vi "03_dosing.vi"() -> ()   [LabVIEW 2024]
uses:
  <vilib>/Utility/error.llb/DialogType.ctl
  <vilib>/Waveform/WDTOps.llb/WDT Waveform to XY Pairs DBL.vi
  <instrlib>/Tektronix DMM40x0 Series/Tektronix DMM40x0 Series.lvlib
panel:
  out "error out":errorcluster
  out "error out 2":errorcluster caption="error out"
  out "STABLE":bool
  in  "Serial Communication":T1={"Baud Rate"=9600, "Parity"=0, "Data Bits"=8, "Stop Bits"=10, "Flow Control"=0} {"Flow Control" items=["None", "XON/XOFF", "RTS/CTS", "XON/XOFF & RTS/CTS", "DTR/DSR", "XON/XOFF & DTR/DSR"]; "Stop Bits" items=["1.0"=10, "1.5"=15, "2.0"=20]; "Data Bits" items=["7"=7, "8"=8]; "Parity" items=["None", "Odd", "Even", "Mark", "Space"]; "Baud Rate" items=["300"=300, "600"=600, "1200"=1200, "2400"=2400, "4800"=4800, "9600"=9600, "19200"=19200]}
  in  "COM PORT (COM2)":refnum<visa-resource-name>
  out "Stability threshold":dbl format="%#_13g"
  out "Waveform Graph":dbl[](graph)
  out "XY pairs":cluster{"x":timestamp, "y":dbl}[](array[cluster]) {"y" format="%0.2f"}
  # "Voltmeter Serial Configuration"
  # "DEFAULT SETTINGS:\n\nTimeout (10000 ms)\nTrigger Count (5000)\nSample Count (1)\n\n****DC VOLTAGE***"
  # "Voltmeter Stability"
  # "0 - Stability threshold not met\n1 - Stability threshold met\n\n\n\n*stability (+/-0.05 mV) of last 15 pts"
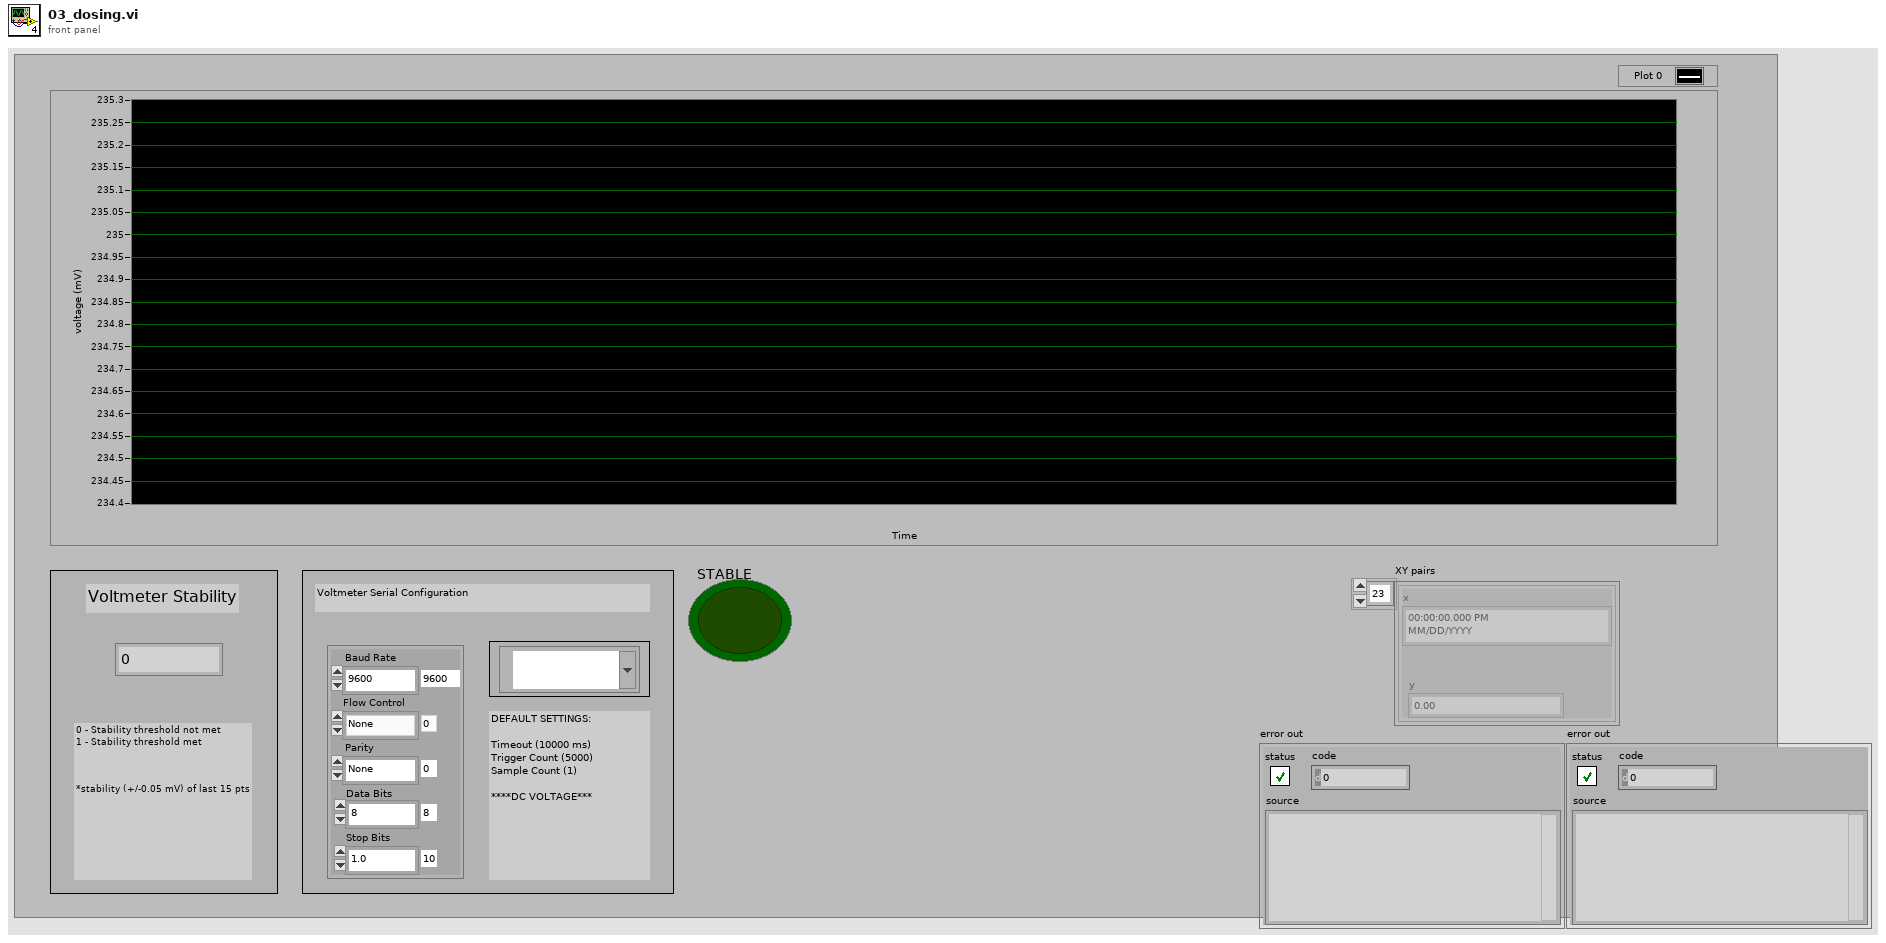
[diagram p1: front panel]
types:
  T1 = cluster{"Baud Rate":u32, "Parity":u16, "Data Bits":u16, "Stop Bits":u16, "Flow Control":u16}
  T2 = typedef "DialogType.ctl" = u16
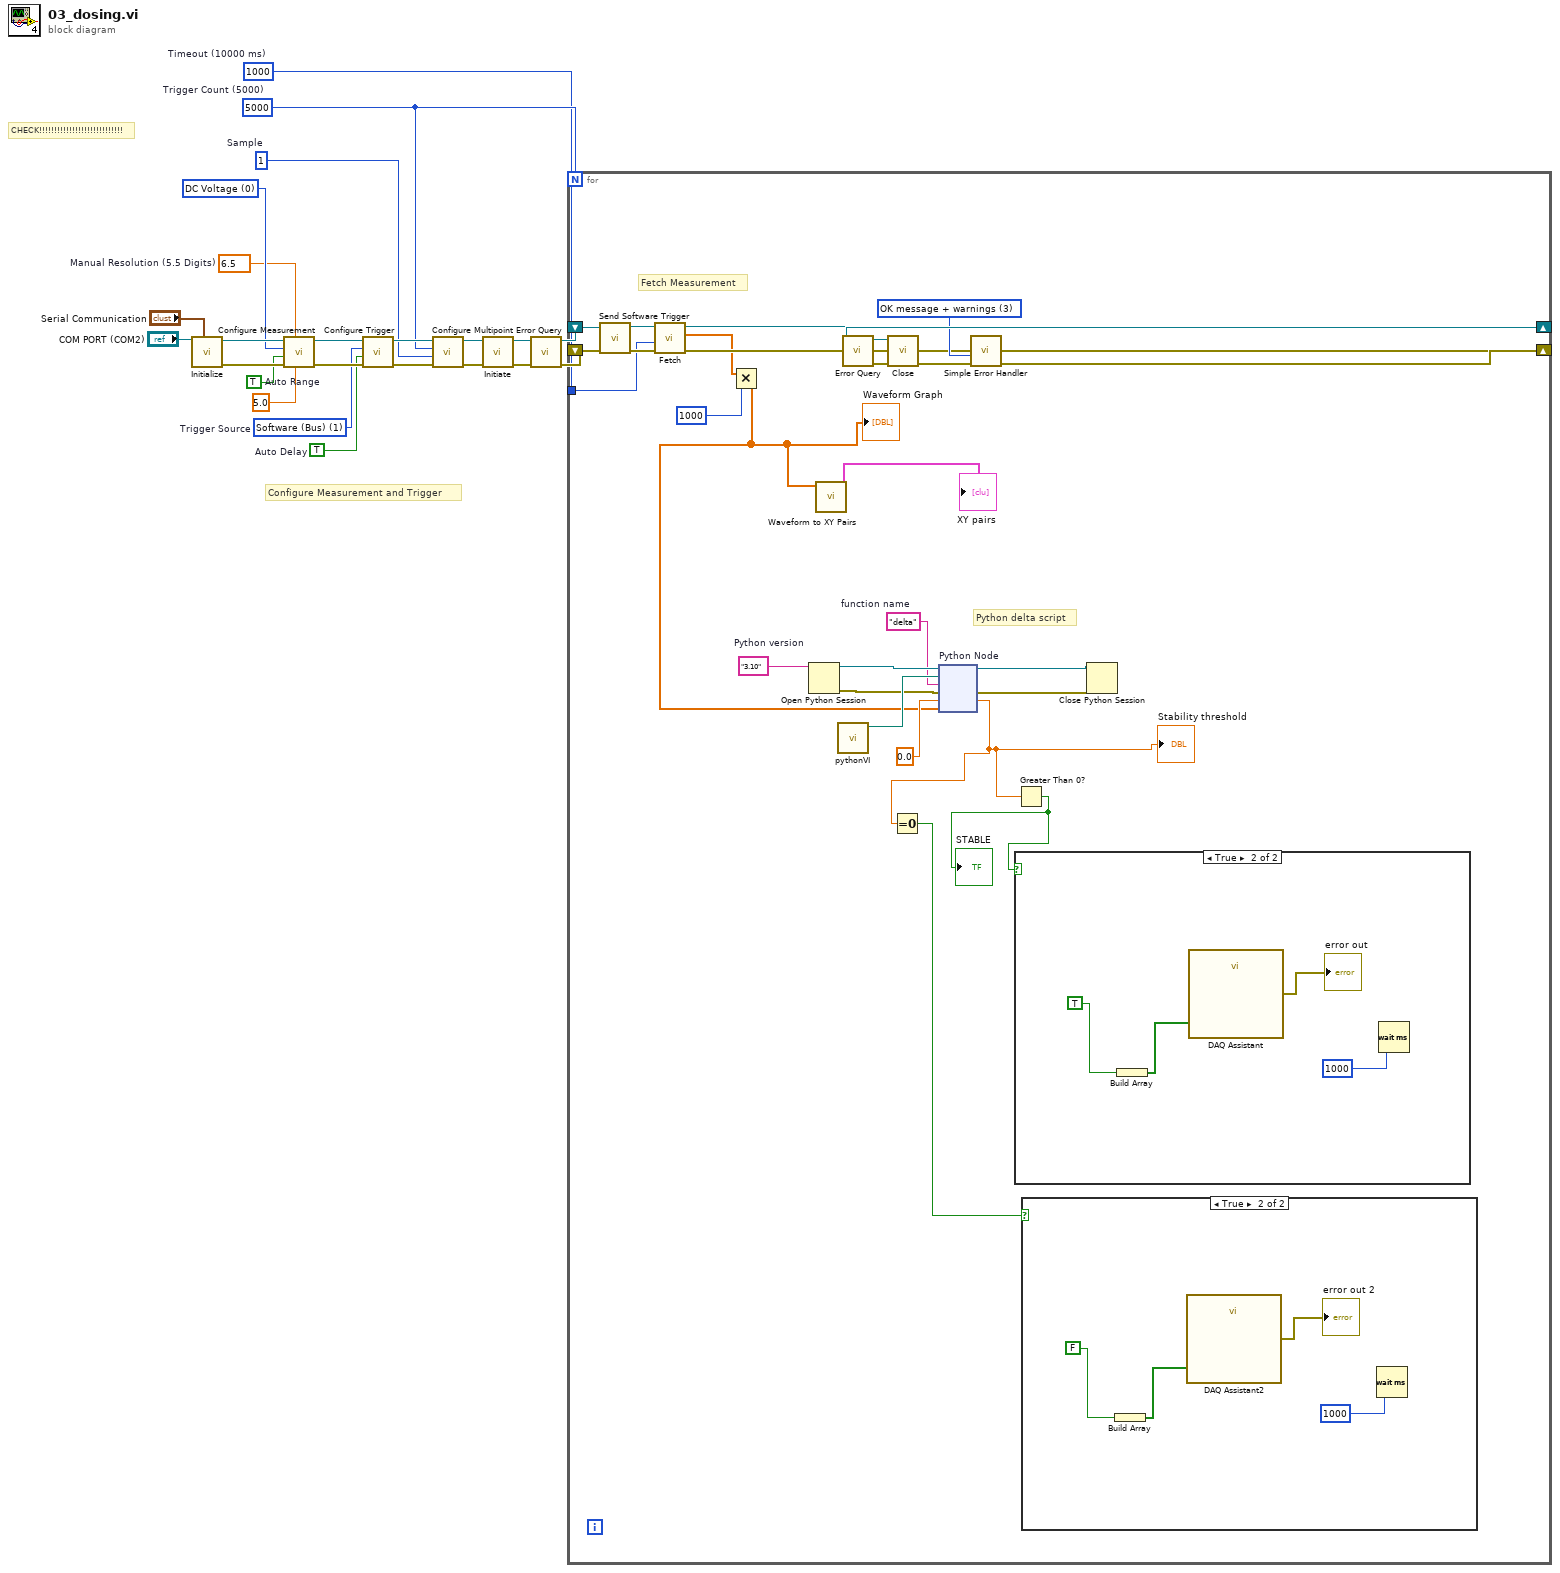
[diagram p0: block diagram]
diagram:
  w10 = u16 0 items=["DC Voltage", "AC Voltage", "2 - Wire Resistance", "4 - Wire Resistance", "DC Current", "AC Current", "Frequency", "Period", "Continuity", "Diode Checking", "Temperature", "Capacitance"] ("Function (0: DC Voltage)")
  w1 = u32 1000  # Timeout (10000 ms)
  w2 = 1  # Sample
  w9 = 5000  # Trigger Count (5000)
  w3 = 6.5 items=["4.5"=4.5, "5.5"=5.5, "6.5"=6.5]  # Manual Resolution (5.5 Digits)
  w11 = TRUE  # Auto Delay
  w12 = u16 1 items=["Immediate", "Software (Bus)", "External"]  # Trigger Source
  w13 = TRUE  # Auto Range
  w16 = T2 3 items=["no dialog", "OK message", "continue or stop message", "OK message + warnings", "continue/stop + warnings"] ("type of dialog (OK msg:1)")
  # "CHECK!!!!!!!!!!!!!!!!!!!!!!!!!!!!"
  # "Configure Measurement and Trigger"
  n1 = call <instrlib>:"Initialize.vi"("Serial Configuration"="Serial Communication", "VISA resource name"="COM PORT (COM2)") -> ("error out"=w28:errorcluster, "VISA resource name out"=w29:refnum<visa-resource-name>)  [unwired: 3 in, 5 out]
  n2 = call <instrlib>:"Configure Measurement.vi"("Manual Range (1.0)"=5.0, "Manual Resolution (5.5 Digits)"=w3, "error in (no error)"=w28, "Auto Range (T:Enable)"=w13, "Function (0: DC Voltage)"=w10, "VISA resource name"=w29) -> ("error out"=w26:errorcluster, "VISA resource name out"=w27:refnum<visa-resource-name>)  [unwired: 4 out]
  n3 = call <instrlib>:"Configure Trigger.vi"("error in (no error)"=w26, "Auto Delay (T: Enable)"=w11, "Trigger Source (0: Immediate)"=w12, "VISA resource name"=w27) -> ("error out"=w24:errorcluster, "VISA resource name out"=w25:refnum<visa-resource-name>)  [unwired: 1 in, 5 out]
  n4 = call <instrlib>:"Configure Multipoint.vi"("error in (no error)"=w24, "Sample Count (1)"=w2, "Trigger Count (1)"=w9, "VISA resource name"=w25) -> ("error out"=w21:errorcluster, "VISA resource name out"=w22:refnum<visa-resource-name>)  [unwired: 6 out]
  n5 = call <instrlib>:"Initiate.vi"("error in (no error)"=w21, "VISA resource name"=w22) -> ("error out"=w8:errorcluster, "VISA resource name out"=w7:refnum<visa-resource-name>)  [unwired: 8 out]
  n6 = call <instrlib>:"Error Query.vi"("error in (no error)"=w8, "VISA resource name"=w7) -> ("error out"=w5:errorcluster, "VISA resource name out"=w6:refnum<visa-resource-name>)  [unwired: 8 out]
  n7 = for {
    N: w9 -> [_]
    shift-right: [w50] -> w18
    shift-left: w5 -> [w46]
    shift-right: [w51] -> w20
    shift-left: w6 -> [w47]
    tunnel: w1 -> [w45]
    w36 = "delta"  # function name
    w34 = "3.10"  # Python version
    # "Python delta script"
    # "Fetch Measurement"
    n8 = call <instrlib>:"Send Software Trigger.vi"("error in (no error)"=w46, "VISA resource name"=w47) -> ("error out"=w48:errorcluster, "VISA resource name out"=w49:refnum<visa-resource-name>)  [unwired: 8 out]
    n9 = call <instrlib>:"Fetch.vi"("error in (no error)"=w48, "Timeout (10000 ms)"=w45, "VISA resource name"=w49) -> ("error out"=w50:errorcluster, "Measurements"=w44:dbl[], "VISA resource name out"=w51:refnum<visa-resource-name>)  [unwired: 6 out]
    n10 = Multiply(x=w44, y=1000) -> (x*y=w33:dbl[])
    "Waveform Graph" <- w33
    n11 = Open Python Session(python version=w34) -> (session out=w40:refnum<k35>, error out=w37:errorcluster)  [unwired: 2 in]
    n12 = call-poly <vilib>:"Waveform to XY Pairs.vi"("waveform in"=w33) -> ("XY pairs"=→"XY pairs":cluster{"x":timestamp, "y":dbl}[])  [unwired: 8 in, 2 out]
    n13 = call "pythonVI.vi"() -> ("appended path"=w41:path)  [unwired: 11 in]
    n14 = node "Python Node"(w40, w41, w36, w37, 0.0, w33) -> (w39:refnum<k35>, w38:errorcluster, w31:dbl)  [unwired: 1 in, 2 out]
    "Stability threshold" <- w31
    n15 = Equal To 0?(x=w31) -> (x = 0?=w30:bool)
    n16 = Greater Than 0?(x=w31) -> (x > 0?=w32:bool)
    "STABLE" <- w32
    n17 = case shown="True" w32 {
      frame False {
      }
      frame True {
        n18 = Build Array(TRUE ("element")) -> (w56:bool[])
        n19 = call "DAQ Assistant"("data"=w56) -> ("error out"=→"error out":errorcluster)  [unwired: 17 in, 1 out]
        n20 = Wait (ms)(milliseconds to wait=u32 1000) -> ()  [unwired: 1 out]
      }
    }
    n21 = case shown="True" w30 {
      frame False {
      }
      frame True {
        n22 = Build Array(FALSE ("element")) -> (w52:bool[])
        n23 = call "DAQ Assistant2"("data"=w52) -> ("error out"=→"error out 2":errorcluster)  [unwired: 17 in, 1 out]
        n24 = Wait (ms)(milliseconds to wait=u32 1000) -> ()  [unwired: 1 out]
      }
    }
    n25 = Close Python Session(session in=w39, error in=w38) -> ()  [unwired: 1 out]
  }
  n26 = call <instrlib>:"Error Query.vi"("error in (no error)"=w18, "VISA resource name"=w20) -> ("error out"=w17:errorcluster, "VISA resource name out"=w19:refnum<visa-resource-name>)  [unwired: 8 out]
  n27 = call <instrlib>:"Close.vi"("error in (no error)"=w17, "VISA resource name"=w19) -> ("error out"=w23:errorcluster)  [unwired: 9 out]
  n28 = call <vilib>:"Simple Error Handler.vi"("type of dialog (OK msg:1)"=w16, "error in (no error)"=w23) -> ()  [unwired: 8 out]
